vi "UpdateData.vi"(1 "Duration Time (ms)":sgl, 4 "Detector Select":enum32{"4 Detectors", "8 Detectors"}(radio)=enum."8 Detectors", 5 "Delay Time":sgl[](array[numeric])) -> (0 "Elapsed Time(s)":sgl, 6 "Intensity Array":sgl[](array[numeric]), 7 "Tau Array":sgl[](array[numeric]), 8 "mean":dbl format="%0.2f", 9 "mean 8":dbl format="%0.2f", 10 "mean 2":dbl format="%0.2f", 11 "mean 7":dbl format="%0.2f", 12 "mean 3":dbl format="%0.2f", 13 "Intensity data":string, 14 "g2 Display":cluster{"Delay Time":sgl[], sgl[]}[](array[cluster]), 15 "mean 4":dbl format="%0.2f", 16 "mean 5":dbl format="%0.2f", 17 "mean 6":dbl format="%0.2f", 18 "tau data":string, 19 "g2 data":string)   [LabVIEW 2016]
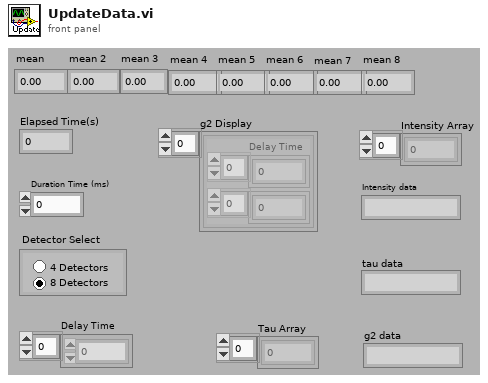
[diagram p1: front panel]
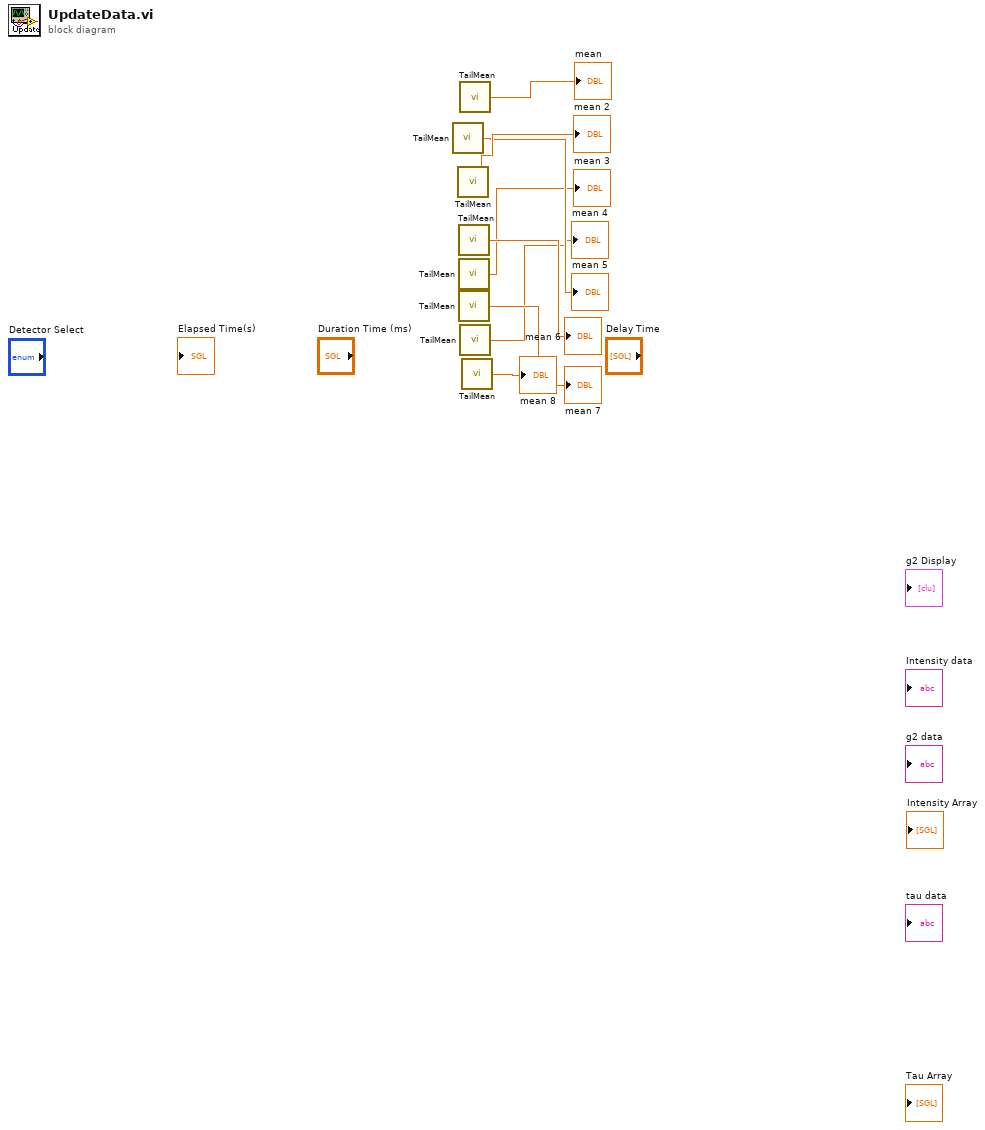
[diagram p0: block diagram]
diagram:
  n1 = call "TailMean.vi"() -> ("mean"=→"mean 5":dbl)  [unwired: 1 in]
  n2 = call "TailMean.vi"() -> ("mean"=→"mean 2":dbl)  [unwired: 1 in]
  n3 = call "TailMean.vi"() -> ("mean"=→"mean 6":dbl)  [unwired: 1 in]
  n4 = call "TailMean.vi"() -> ("mean"=→"mean 3":dbl)  [unwired: 1 in]
  n5 = call "TailMean.vi"() -> ("mean"=→"mean 7":dbl)  [unwired: 1 in]
  n6 = call "TailMean.vi"() -> ("mean"=→"mean":dbl)  [unwired: 1 in]
  n7 = call "TailMean.vi"() -> ("mean"=→"mean 4":dbl)  [unwired: 1 in]
  n8 = call "TailMean.vi"() -> ("mean"=→"mean 8":dbl)  [unwired: 1 in]
